vi "switch_GD.vi"(0 "Gd switches":string, 1 "Node":string, 2 "event time":string="0.023560", 3 "Event type":string="BCG") -> (7 "updated switch":string)   [LabVIEW 2020]
uses:
  <vilib>/regexp/Match Regular Expression.xnode
panel:
  out "after substring":string
  out "substring":string
  out "GD number":string
  out "Result":string
  out "after match":string
  out "whole match":string
  out "before match":string
  out "Event switches":string caption="Result"
  in  "Evento?":bool
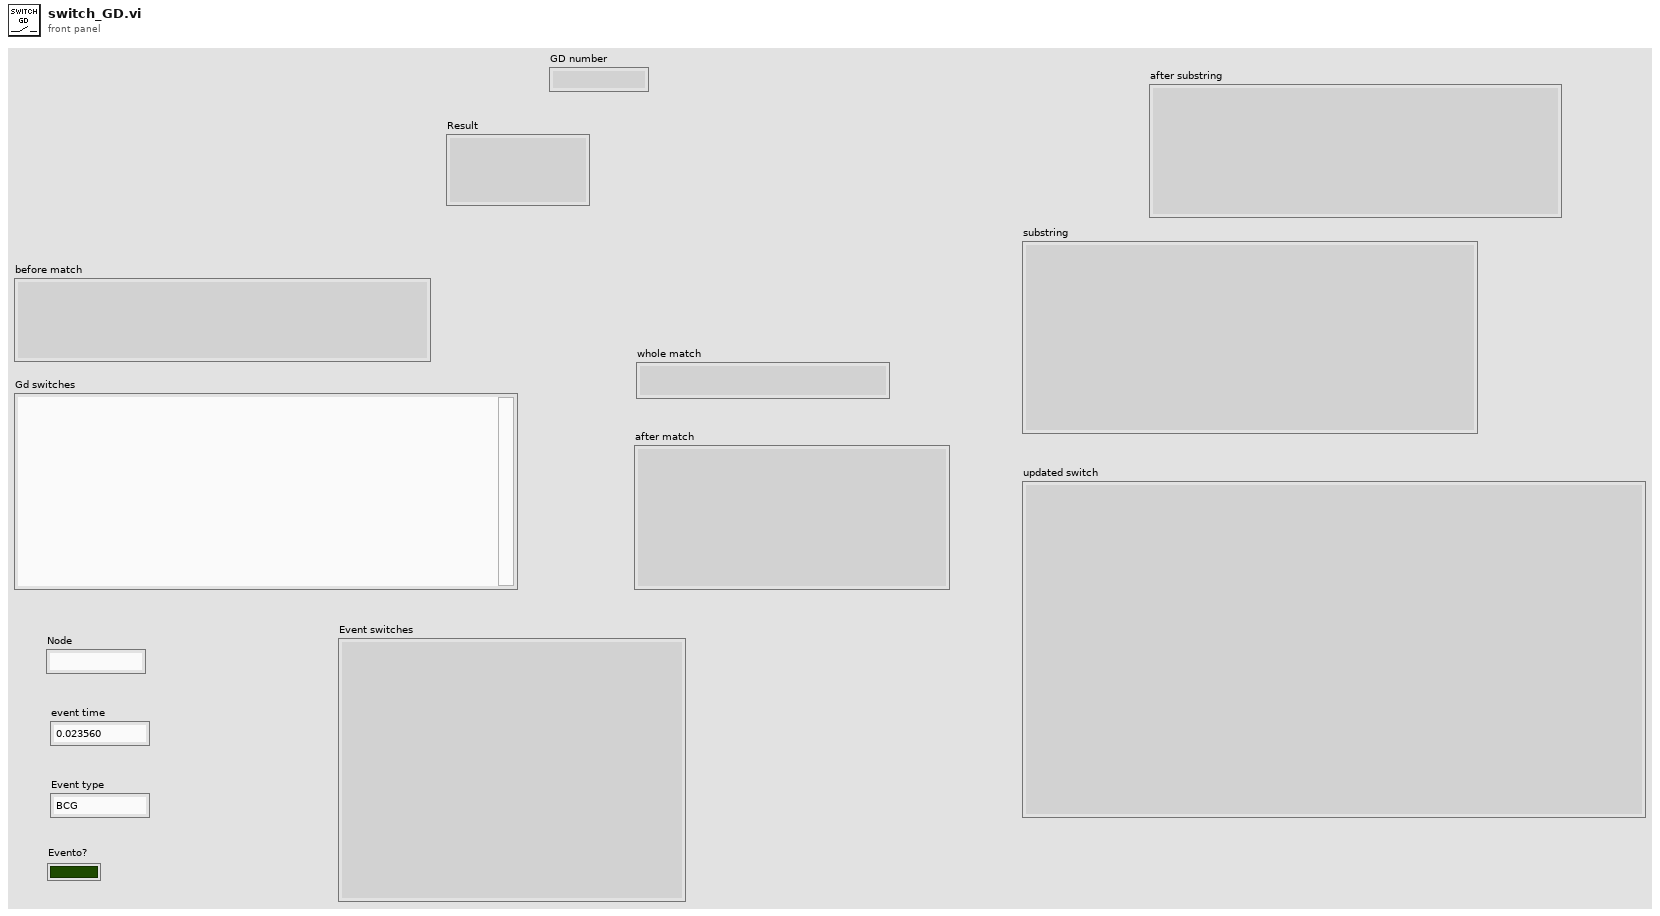
[diagram p1: front panel]
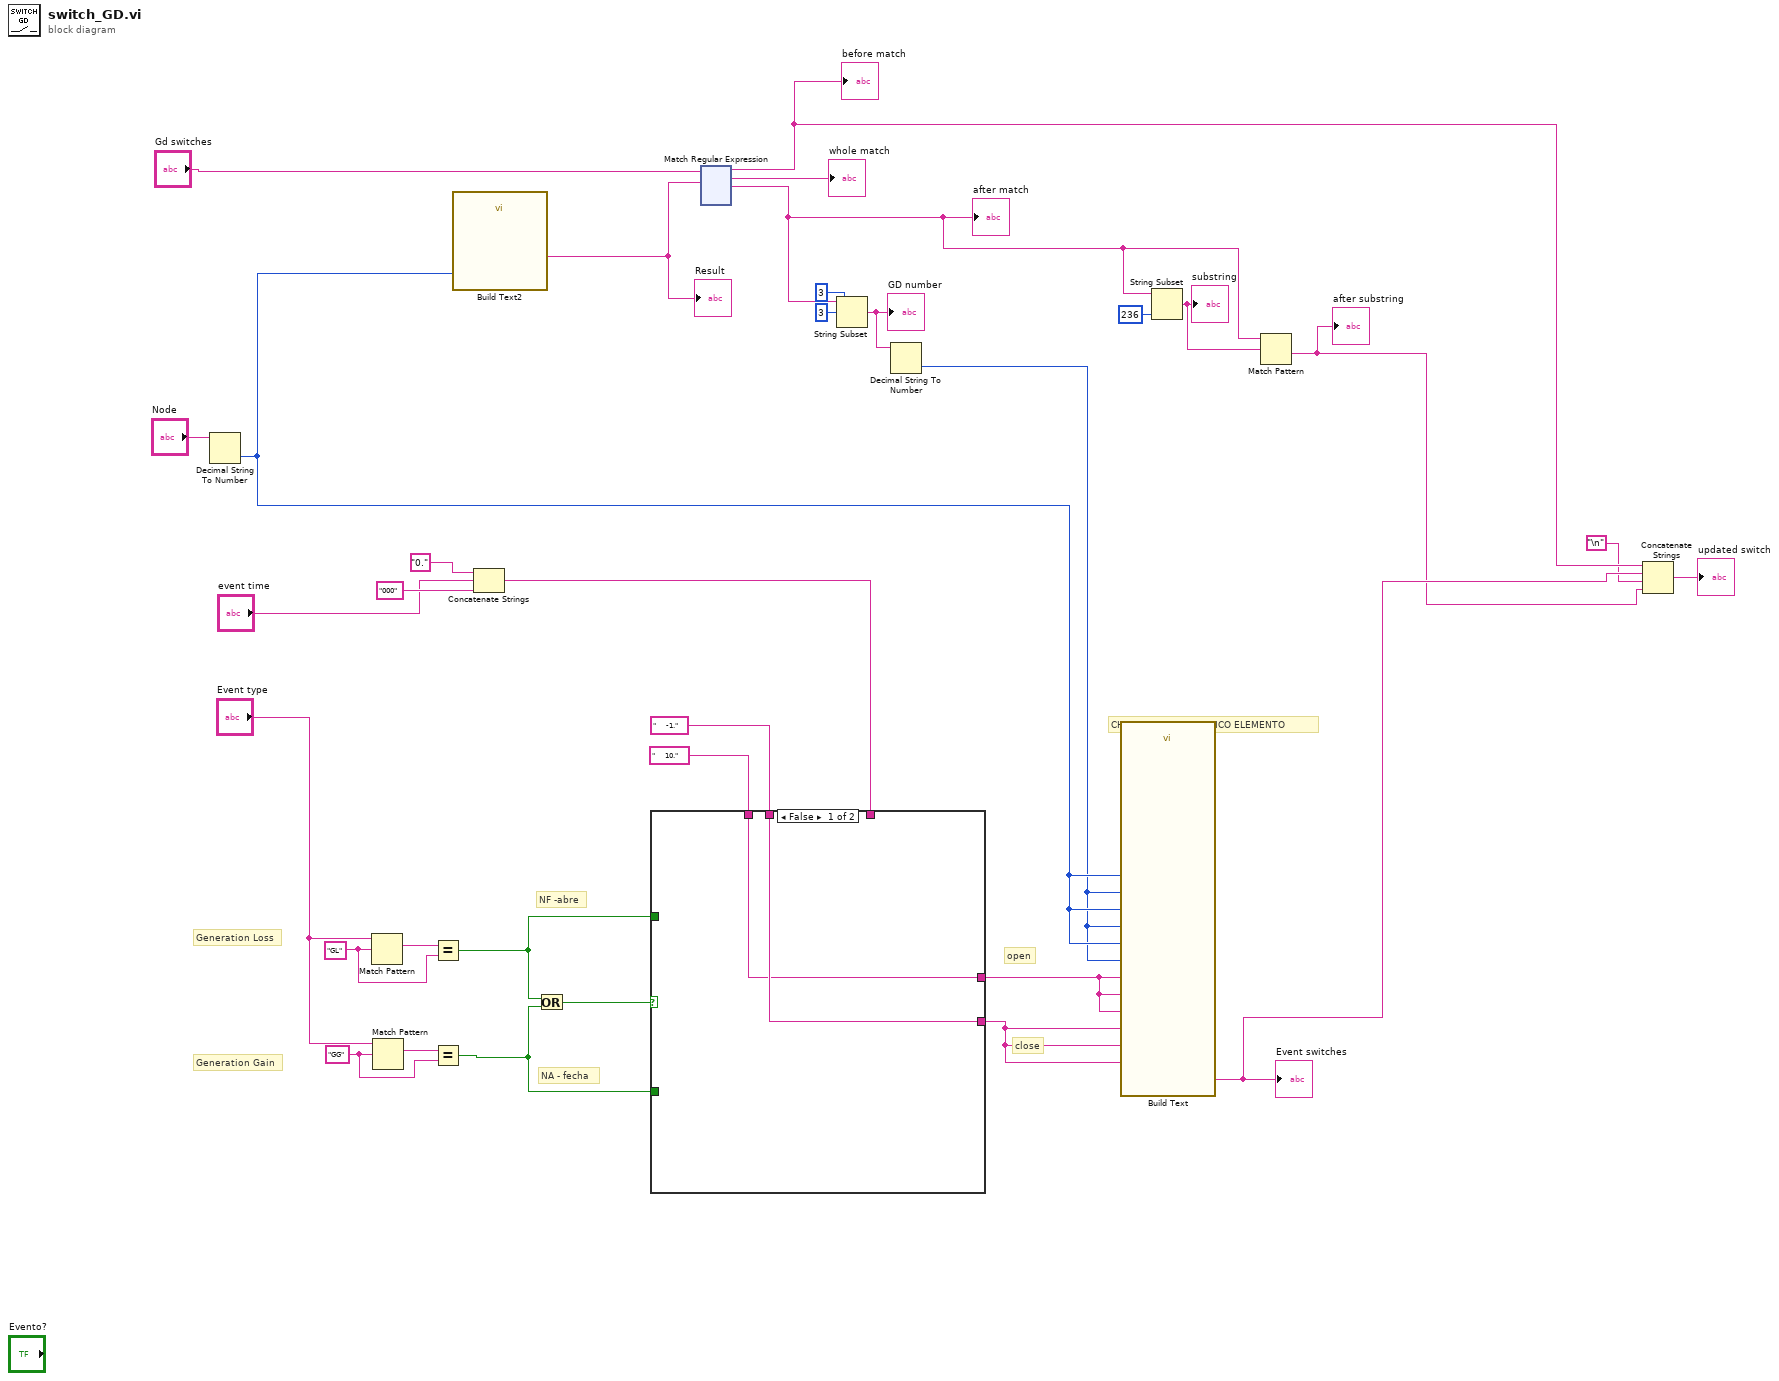
[diagram p0: block diagram]
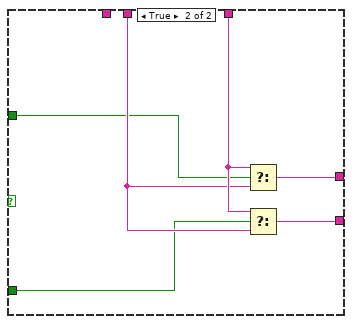
[diagram p2: hidden frame]
diagram:
  w27 = "GL" ("regular expression")
  w28 = "GG" ("regular expression")
  # "close"
  # "open"
  # "CHAVEAMENTO DE UNICO ELEMENTO"
  # "NA - fecha"
  # "NF -abre"
  # "Generation Gain"
  # "Generation Loss"
  n1 = Decimal String To Number(string="Node") -> (number=w13:i32)  [unwired: 2 in, 1 out]
  n2 = Match Pattern(string="Event type", regular expression=w27) -> (match substring=w26:string)  [unwired: 1 in, 3 out]
  n3 = Match Pattern(string="Event type", regular expression=w28) -> (match substring=w31:string)  [unwired: 1 in, 3 out]
  n4 = Equal?(x=w26, y=w27) -> (x = y?=w19:bool)
  n5 = Equal?(x=w31, y=w28) -> (x = y?=w18:bool)
  n6 = call "Build Text2"("node"=w13) -> ("Result"=w15:string)  [unwired: 13 in, 1 out]
  "Result" <- w15
  n7 = Concatenate Strings("0." ("string"), "event time", "000" ("string")) -> (w22:string)
  n8 = Or(x=w19, y=w18) -> (x .or. y?=w30:bool)
  n9 = case shown="False" w30 {
    tunnel: w22 -> [_ w41]
    tunnel: "     -1." -> [w35 w38]
    tunnel: "     10." -> [w34 _]
    tunnel: [w35 w39] -> w20
    tunnel: [w34 w40] -> w21
    tunnel: w18 -> [_ w36]
    tunnel: w19 -> [_ w37]
    frame False {
    }
    frame True {
      n10 = Select(t=w41, s=w37, f=w38) -> (s? t:f=w40:string)
      n11 = Select(t=w41, s=w36, f=w38) -> (s? t:f=w39:string)
    }
  }
  n12 = xnode "Match Regular Expression"("input string"="Gd switches", "regular expression"=w15) -> ("before match"=w8:string, "whole match"=→"whole match":string, "after match"=w3:string)  [unwired: 4 in, 2 out]
  "before match" <- w8
  "after match" <- w3
  n13 = String Subset(string=w3, offset (0)=3, length (rest)=3 ("length (rest)")) -> (substring=w10:string)
  "GD number" <- w10
  n14 = Decimal String To Number(string=w10) -> (number=w9:i32)  [unwired: 2 in, 1 out]
  n15 = call "Build Text"("inA"=w13, "inA_2"=w9, "time_close_A"=w20, "time_open_A"=w21, "inB"=w13, "inB_2"=w9, "time_close_B"=w20, "time_open_B"=w21, "inC"=w13, "inC_2"=w9, "time_close_C"=w20, "time_open_C"=w21) -> ("Result"=w6:string)  [unwired: 14 in, 1 out]
  "Event switches" <- w6
  n16 = String Subset(string=w3, length (rest)=236 ("length (rest)")) -> (substring=w2:string)  [unwired: 1 in]
  "substring" <- w2
  n17 = Match Pattern(string=w3, regular expression=w2) -> (after substring=w1:string)  [unwired: 1 in, 3 out]
  "after substring" <- w1
  n18 = Concatenate Strings(w8, w6, "\n", w1) -> (→"updated switch":string)
